vi "Read Swipe XZ Vector.vi"   [LabVIEW 2011, in "LVH-Leap.lvlib"]
uses:
  LVH-Leap.lvlib
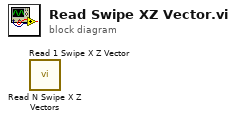
[diagram p0: block diagram]
diagram:
  n1 = call "Read N Swipe X Z Vectors.vi"() -> ()  [unwired: 9 in, 3 out]
  n2 = call "Read 1 Swipe X Z Vector.vi"() -> ()  [unwired: 8 in, 4 out]
